vi "Wait.vi"(0 "Battery Detect Voltage (0V)":dbl format="%#.6g", 1 "VISA resource name":refnum<visa-resource-name>, 3 "Path":path, 4 "DAQmx Task Name":refnum<k21>, 5 "Wait time":dbl, 11 "Task error in":errorcluster, 12 "Visa error in (no error)":errorcluster caption="error in (no error)") -> (6 "VISA resource name out":refnum<visa-resource-name>, 8 "Filename Out":path, 9 "WaitElapsed Time (s)":dbl caption="Elapsed Time (s)", 10 "task out":refnum<k21>, 14 "Task error out":errorcluster, 15 "Visa error out":errorcluster)   [LabVIEW 2020]
uses:
  <vilib>/DAQmx/read.llb/DAQmx Read (Analog 1D DBL NChan 1Samp).vi
  <vilib>/DAQmx/miscellaneous.llb/DAQmx Fill In Error Info.vi
  <instrlib>/NH Research Regenerative Test Series/Public/Data/Read (Ave Current).vi
  <instrlib>/NH Research Regenerative Test Series/Public/Data/Low Level/Fetch (Ave Voltage).vi
  <instrlib>/NH Research Regenerative Test Series/Public/Data/Low Level/Fetch (Ave True Power).vi
  <instrlib>/NH Research Regenerative Test Series/NH Research Regenerative Test Series.lvlib
panel:
  out "Ave Current (A)":dbl
  out "Ave Voltage (V)":dbl
  out "Ave True Power (W)":dbl
  out "Status Byte Register":T1
  in  "Logical Instrument Number":u32=1
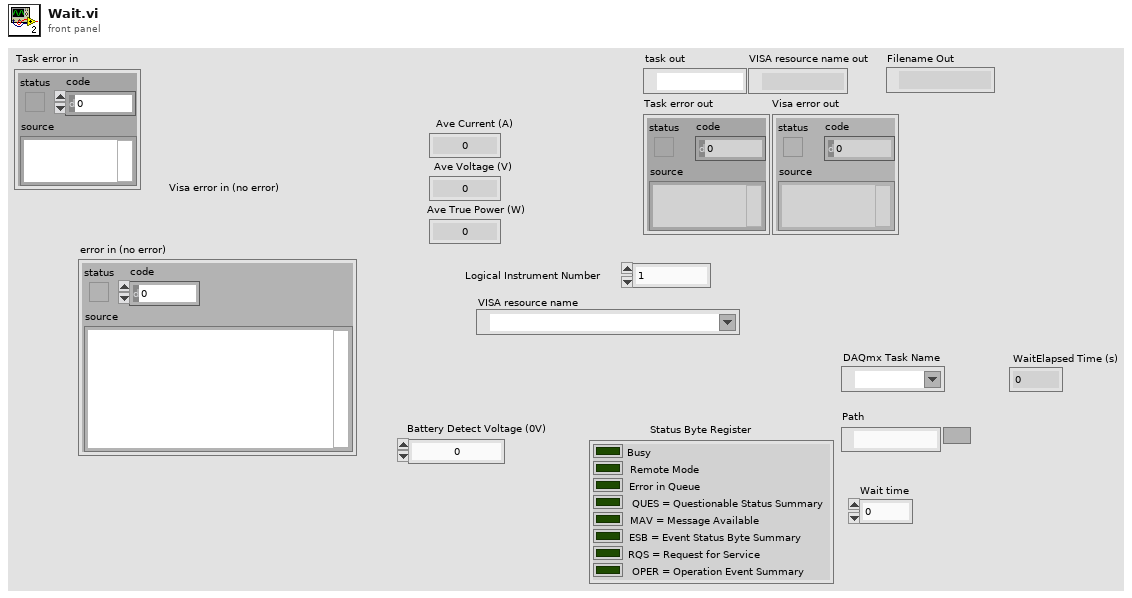
[diagram p1: front panel]
types:
  T1 = cluster{"Busy":bool, "Remote Mode":bool, "Error in Queue":bool, "QUES = Questionable Status Summary":bool, "MAV = Message Available":bool, "ESB = Event Status Byte Summary":bool, "RQS = Request for Service":bool, "OPER = Operation Event Summary":bool}
  T2 = cluster{"data[0]":dbl, "data[1]":dbl, "data[2]":dbl, "data[3]":dbl, "data[4]":dbl, "data[5]":dbl, "data[6]":dbl, "data[7]":dbl, "data[8]":dbl}
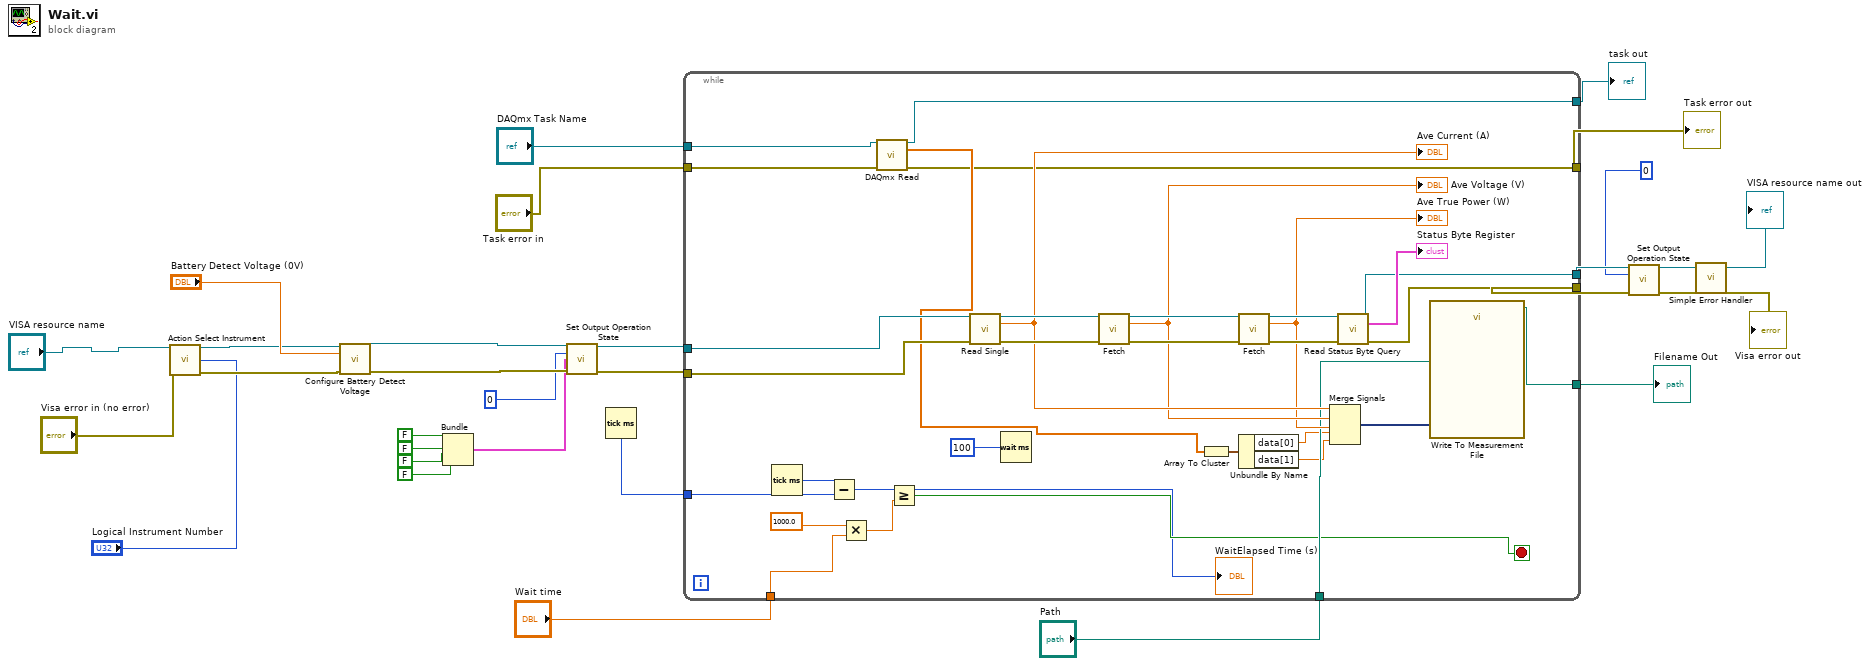
[diagram p0: block diagram]
diagram:
  n1 = call <instrlib>:"Action Select Instrument.vi"("VISA resource name"="VISA resource name", "Logical Instrument Number"="Logical Instrument Number", "error in (no error)"="Visa error in (no error)") -> ("VISA resource name out"=w28:refnum<visa-resource-name>, "error out"=w27:errorcluster)  [unwired: 11 in]
  n2 = call <vilib>:"Configure Battery Detect Voltage.vi"("VISA resource name"=w28, "Battery Detect Voltage (0V)"="Battery Detect Voltage (0V)", "error in (no error)"=w27) -> ("VISA resource name out"=w26:refnum<visa-resource-name>, "error out"=w25:errorcluster)  [unwired: 11 in]
  n3 = Bundle(FALSE, FALSE, FALSE, FALSE) -> (w12:cluster{bool, bool, bool, bool})  [unwired: 1 in]
  n4 = call <vilib>:"Set Output Operation State.vi"("VISA resource name"=w26, "Mode (0: Off)"=0, "Enable"=w12, "error in (no error)"=w25) -> ("VISA resource name out"=w21:refnum<visa-resource-name>, "error out"=w20:errorcluster)  [unwired: 10 in]
  n5 = Tick Count (ms)() -> (millisecond timer value=w8:u32)
  n6 = while {
    tunnel: w21 -> [w55]
    tunnel: w20 -> [w54]
    tunnel: [w52] -> w24
    tunnel: [w51] -> w23
    tunnel: "Wait time" -> [w36]
    tunnel: "Path" -> [w47]
    tunnel: "DAQmx Task Name" -> [w46]
    tunnel: w8 -> [w38]
    tunnel: [w33] -> w7
    tunnel: [w32] -> w6
    tunnel: "Task error in" -> [w31]
    tunnel: [w30] -> w1
    stop <- w39 stop-if-true
    n7 = Tick Count (ms)() -> (millisecond timer value=w40:u32)
    n8 = Subtract(x=w40, y=w38) -> (x-y=w37:u32)
    "WaitElapsed Time (s)" <- w37
    n9 = Multiply(x=1000.0, y=w36) -> (x*y=w34:dbl)
    n10 = call-poly <vilib>:"DAQmx Read.vi"("task/channels in"=w46, "error in"=w31) -> ("task out"=w32:refnum<k21>, "data"=w45:dbl[], "error out"=w33:errorcluster)  [unwired: 11 in]
    n11 = Greater Or Equal?(x=w37, y=w34) -> (x >= y?=w39:bool)
    n12 = call-poly <instrlib>:"Read Single.vi"("VISA resource name"=w55, "error in (no error)"=w54) -> ("VISA resource name out"=w60:refnum<visa-resource-name>, "Ave Current (A)"=w50:dbl, "error out"=w61:errorcluster)  [unwired: 11 in]
    "Ave Current (A)" <- w50
    n13 = Wait (ms)(milliseconds to wait=100) -> ()  [unwired: 1 out]
    n14 = call-poly <instrlib>:"Fetch.vi"("VISA resource name"=w60, "error in (no error)"=w61) -> ("VISA resource name out"=w59:refnum<visa-resource-name>, "Ave Voltage (V)"=w49:dbl, "error out"=w58:errorcluster)  [unwired: 11 in]
    "Ave Voltage (V)" <- w49
    n15 = Array To Cluster(array=w45) -> (cluster=w44:T2)
    n16 = call-poly <instrlib>:"Fetch.vi"("VISA resource name"=w59, "error in (no error)"=w58) -> ("VISA resource name out"=w57:refnum<visa-resource-name>, "Ave True Power (W)"=w48:dbl, "error out"=w56:errorcluster)  [unwired: 11 in]
    "Ave True Power (W)" <- w48
    n17 = Unbundle By Name(w44) -> ("data[0]"=w43:dbl, "data[1]"=w42:dbl)
    n18 = Merge Signals "Merge Signals"(w50, w49, w48, w43, w42) -> (w62:dynamicdata)
    n19 = call <instrlib>:"Read Status Byte Query.vi"("VISA resource name"=w57, "error in (no error)"=w56) -> ("VISA resource name out"=w52:refnum<visa-resource-name>, "Status Byte Register"=→"Status Byte Register":T1, "error out"=w51:errorcluster)  [unwired: 11 in]
    n20 = call "Write To Measurement File"("Signals"=w62, "Filename"=w47) -> ("Filename Out"=w30:path)  [unwired: 15 in, 2 out]
  }
  "Task error out" <- w7
  "task out" <- w6
  "Filename Out" <- w1
  n21 = call <vilib>:"Set Output Operation State.vi"("VISA resource name"=w24, "Mode (0: Off)"=0, "error in (no error)"=w23) -> ("VISA resource name out"=→"VISA resource name out":refnum<visa-resource-name>, "error out"=→"Visa error out":errorcluster)  [unwired: 11 in]
  n22 = call <vilib>:"Simple Error Handler.vi"() -> ()  [unwired: 5 in, 5 out]
